vi "HelloWorld.vi"() -> ()   [LabVIEW 2020]
panel:
  out "Waveform Graph":dbl[](graph)
  in  "stop 2":bool
  out "Waveform Chart":dbl(graph)
  out "Numeric 5":dbl
  out "Numeric 4":dbl
  in  "Temp (F) 2":dbl(slide) scale=0.0..200.0
  in  "stop":bool
  in  "Boolean":bool
  out "Numeric 3":dbl
  out "Numeric 2":dbl
  in  "Temp (F)":dbl(slide) scale=0.0..200.0
  out "Temp (C)":dbl(slide) scale=0.0..100.0
  out "String 2":string
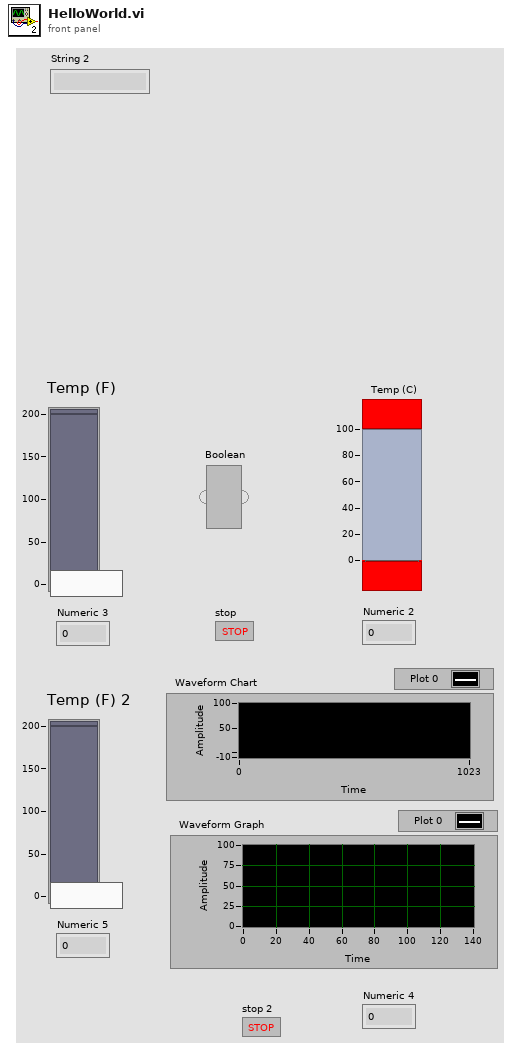
[diagram p1: front panel]
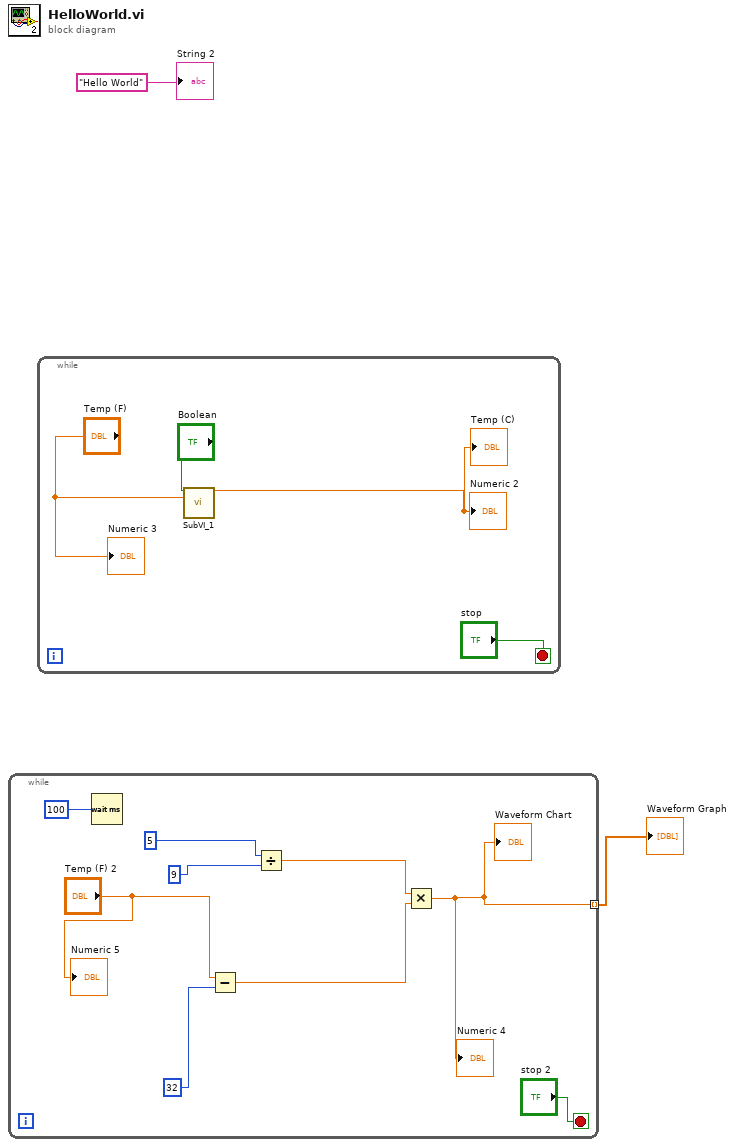
[diagram p0: block diagram]
diagram:
  n1 = while {
    tunnel: [w3] -> w1 mode=indexing
    stop <- "stop 2" stop-if-true
    n2 = Wait (ms)(milliseconds to wait=u32 100 ("millisecond timer value")) -> ()  [unwired: 1 out]
    n3 = Subtract(x="Temp (F) 2", y=32) -> (x-y=w8:dbl)
    n4 = Divide(x=5, y=9) -> (x/y=w9:dbl)
    n5 = Multiply(x=w9, y=w8) -> (x*y=w3:dbl)
    "Numeric 4" <- w3
    "Waveform Chart" <- w3
    "Numeric 5" <- "Temp (F) 2"
  }
  "Waveform Graph" <- w1
  n6 = while {
    stop <- "stop" stop-if-true
    n7 = call "SubVI_1.vi"("Boolean"="Boolean", "Temp (F)"="Temp (F)") -> ("Numeric"=→"Temp (C)" →"Numeric 2":dbl)  [unwired: 13 in]
    "Numeric 3" <- "Temp (F)"
  }
  "String 2" <- "Hello World"
